vi "SetNavigationInProgress.vi"(8 "error in (no error)":errorcluster, 10 "navigation in progress":bool, 11 "AbstractWorldMap in":refnum<class "NI_Robotics_AbstractWorldMap.lvclass">) -> (0 "error out":errorcluster, 3 "AbstractWorldMap out":refnum<class "NI_Robotics_AbstractWorldMap.lvclass">)   [LabVIEW 2017, in "NI_Robotics_AbstractWorldMap.lvclass"]
uses:
  <vilib>/robotics/Navigation/shared/WorldMap/AbstractWorldMap/NI_Robotics_AbstractWorldMap.lvclass
  <vilib>/robotics/Navigation/shared/WorldMap/AbstractWorldMap/NI_Robotics_AbstractWorldMap.lvclass/NI_Robotics_AbstractWorldMap.ctl
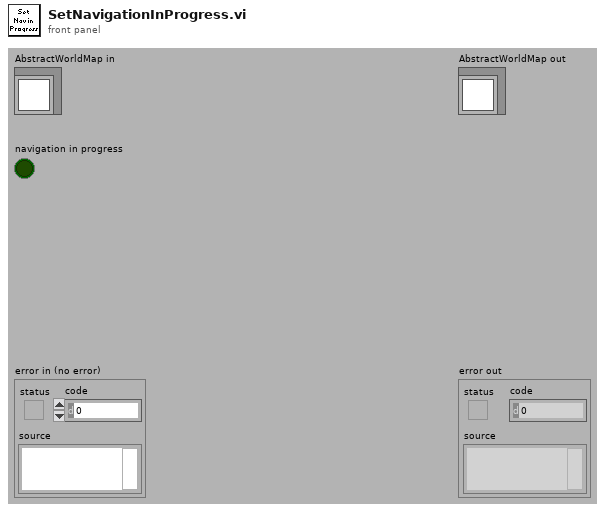
[diagram p1: front panel]
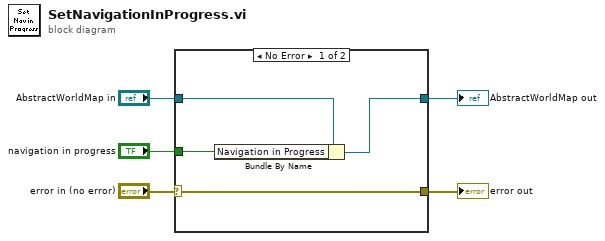
[diagram p0: block diagram]
diagram:
  n1 = case shown="No Error" "error in (no error)" {
    selector: "error in (no error)" -> [w9 w10]
    tunnel: [w9 w10] -> w4
    tunnel: [w7 w11] -> w2
    tunnel: "AbstractWorldMap in" -> [w8 w11]
    tunnel: "navigation in progress" -> [w6 _]
    frame No Error {
      n2 = Bundle By Name(cluster=w8, "Navigation in Progress"=w6) -> (w7:refnum<class "NI_Robotics_AbstractWorldMap.lvclass">)
    }
    frame Error {
    }
  }
  "error out" <- w4
  "AbstractWorldMap out" <- w2
